vi "Get 4 Tables BY DP.vi"(0 "Air Pressure [psia]":dbl, 3 "Dew Point [DegF]":dbl) -> (1 "Pressure Z":dbl=53.278814892593125, 4 "DP Z":dbl, 5 "HP Higher DP Psych Table":dbl[][](array[numeric])=[[6500.0, 11.55684946, 0.0, 0.0, 0.0, 0.0, 0.0, 0.0, 0.0, 5.0], [6500.0, 11.55684946, 5.0, 5.0, 100.0, 0.001292913, 9.050389509, 14.92783844, 2.574650733, 5.0], [6500.0, 11.55684946, 10.0, 8.763538956, 77.60281671, 0.001292913, 9.050389509, 15.08846683, 3.777521, 5.0], [6500.0, 11.55684946, 15.0, 12.36490821, 60.54642502, 0.001292913, 9.050389509, 15.24909521, 4.980391266, 5.0], [6500.0, 11.55684946, 20.0, 15.80209708, 47.4855805, 0.001292913, 9.050389509, 15.4097236, 6.183261533, 5.0], [6500.0, 11.55684946, 25.0, 19.0756876, 37.43077436, 0.001292913, 9.050389509, 15.57035199, 7.386131799, 5.0], [6500.0, 11.55684946, 30.0, 22.18850798, 29.64995401, 0.001292913, 9.050389509, 15.73098037, 8.589002065, 5.0], [6500.0, 11.55684946, 35.0, 25.14521247, 23.98042946, 0.001292913, 9.050389509, 15.89160876, 9.791872332, 5.0], [6500.0, 11.55684946, 40.0, 27.95183421, 19.69610149, 0.001292913, 9.050389509, 16.05223714, 10.9947426, 5.0], [6500.0, 11.55684946, 45.0, 30.61535932, 16.2482458, 0.001292913, 9.050389509, 16.21286553, 12.19761286, 5.0], [6500.0, 11.55684946, 50.0, 33.21581881, 13.4609987, 0.001292913, 9.050389509, 16.37349392, 13.40048313, 5.0], [6500.0, 11.55684946, 55.0, 35.78456941, 11.19790107, 0.001292913, 9.050389509, 16.5341223, 14.6033534, 5.0], [6500.0, 11.55684946, 60.0, 38.24289128, 9.352562028, 0.001292913, 9.050389509, 16.69475069, 15.80622366, 5.0], [6500.0, 11.55684946, 65.0, 40.59668627, 7.841647488, 0.001292913, 9.050389509, 16.85537907, 17.00909393, 5.0], [6500.0, 11.55684946, 70.0, 42.851757, 6.599588278, 0.001292913, 9.050389509, 17.01600746, 18.2119642, 5.0], [6500.0, 11.55684946, 75.0, 45.01373336, 5.574566408, 0.001292913, 9.050389509, 17.17663585, 19.41483446, 5.0], [6500.0, 11.55684946, 80.0, 47.08801848, 4.725456286, 0.001292913, 9.050389509, 17.33726423, 20.61770473, 5.0], [6500.0, 11.55684946, 85.0, 49.07976369, 4.019482866, 0.001292913, 9.050389509, 17.49789262, 21.820575, 5.0], [6500.0, 11.55684946, 90.0, 50.99384196, 3.430420591, 0.001292913, 9.050389509, 17.65852101, 23.02344526, 5.0], [6500.0, 11.55684946, 95.0, 52.83484458, 2.937202158, 0.001292913, 9.050389509, 17.81914939, 24.22631553, 5.0], [6500.0, 11.55684946, 100.0, 54.60708072, 2.522839263, 0.001292913, 9.050389509, 17.97977778, 25.42918579, 5.0], [6500.0, 11.55684946, 105.0, 56.31458155, 2.173581867, 0.001292913, 9.050389509, 18.14040616, 26.63205606, 5.0], [6500.0, 11.55684946, 110.0, 57.9611144, 1.878260621, 0.001292913, 9.050389509, 18.30103455, 27.83492633, 5.0], [6500.0, 11.55684946, 115.0, 59.55019028, 1.62777051, 0.001292913, 9.050389509, 18.46166294, 29.03779659, 5.0], [6500.0, 11.55684946, 120.0, 61.08508025, 1.414663823, 0.001292913, 9.050389509, 18.62229132, 30.24066686, 5.0]], 6 "HP Lower DP Psych Table":dbl[][](array[numeric])=[[6500.0, 11.55684946, 0.0, 8.36519e-16, 100.0, 0.000997316, 6.981212001, 14.76020634, 1.058152276, 0.0], [6500.0, 11.55684946, 5.0, 3.963707944, 77.17374703, 0.000997316, 6.981212001, 14.92075855, 2.260366318, 0.0], [6500.0, 11.55684946, 10.0, 7.771498018, 59.88900146, 0.000997316, 6.981212001, 15.08131075, 3.462580359, 0.0], [6500.0, 11.55684946, 15.0, 11.41785035, 46.72594488, 0.000997316, 6.981212001, 15.24186295, 4.664794401, 0.0], [6500.0, 11.55684946, 20.0, 14.90004443, 36.64640178, 0.000997316, 6.981212001, 15.40241516, 5.867008442, 0.0], [6500.0, 11.55684946, 25.0, 18.218017, 28.88673111, 0.000997316, 6.981212001, 15.56296736, 7.069222484, 0.0], [6500.0, 11.55684946, 30.0, 21.37405669, 22.8819805, 0.000997316, 6.981212001, 15.72351957, 8.271436525, 0.0], [6500.0, 11.55684946, 35.0, 24.37240393, 18.50659597, 0.000997316, 6.981212001, 15.88407177, 9.473650567, 0.0], [6500.0, 11.55684946, 40.0, 27.21878765, 15.20021954, 0.000997316, 6.981212001, 16.04462398, 10.67586461, 0.0], [6500.0, 11.55684946, 45.0, 29.9200054, 12.53938011, 0.000997316, 6.981212001, 16.20517618, 11.87807865, 0.0], [6500.0, 11.55684946, 50.0, 32.51301876, 10.38835708, 0.000997316, 6.981212001, 16.36572838, 13.08029269, 0.0], [6500.0, 11.55684946, 55.0, 35.11238388, 8.641839847, 0.000997316, 6.981212001, 16.52628059, 14.28250673, 0.0], [6500.0, 11.55684946, 60.0, 37.59965819, 7.217722561, 0.000997316, 6.981212001, 16.68683279, 15.48472077, 0.0], [6500.0, 11.55684946, 65.0, 39.98076757, 6.051693196, 0.000997316, 6.981212001, 16.847385, 16.68693482, 0.0], [6500.0, 11.55684946, 70.0, 42.26156139, 5.093149563, 0.000997316, 6.981212001, 17.0079372, 17.88914886, 0.0], [6500.0, 11.55684946, 75.0, 44.44773195, 4.302101778, 0.000997316, 6.981212001, 17.1684894, 19.0913629, 0.0], [6500.0, 11.55684946, 80.0, 46.54475421, 3.64681168, 0.000997316, 6.981212001, 17.32904161, 20.29357694, 0.0], [6500.0, 11.55684946, 85.0, 48.55785849, 3.101985539, 0.000997316, 6.981212001, 17.48959381, 21.49579098, 0.0], [6500.0, 11.55684946, 90.0, 50.49199835, 2.647384109, 0.000997316, 6.981212001, 17.65014602, 22.69800502, 0.0], [6500.0, 11.55684946, 95.0, 52.35184609, 2.266748963, 0.000997316, 6.981212001, 17.81069822, 23.90021906, 0.0], [6500.0, 11.55684946, 100.0, 54.14179034, 1.946969591, 0.000997316, 6.981212001, 17.97125043, 25.10243311, 0.0], [6500.0, 11.55684946, 105.0, 55.86593869, 1.677434572, 0.000997316, 6.981212001, 18.13180263, 26.30464715, 0.0], [6500.0, 11.55684946, 110.0, 57.52813184, 1.4495241, 0.000997316, 6.981212001, 18.29235483, 27.50686119, 0.0], [6500.0, 11.55684946, 115.0, 59.13194983, 1.256211495, 0.000997316, 6.981212001, 18.45290704, 28.70907523, 0.0], [6500.0, 11.55684946, 120.0, 60.6807286, 1.09174908, 0.000997316, 6.981212001, 18.61345924, 29.91128927, 0.0]], 7 "LP Higher DP Psych Table":dbl[][](array[numeric])=[[7000.0, 11.3399368, 0.0, 0.0, 0.0, 0.0, 0.0, 0.0, 0.0, 5.0], [7000.0, 11.3399368, 5.0, 5.0, 100.0, 0.001317696, 9.223874019, 15.21398618, 2.601001048, 5.0], [7000.0, 11.3399368, 10.0, 8.746163989, 77.60281671, 0.001317696, 9.223874019, 15.37769361, 3.803926334, 5.0], [7000.0, 11.3399368, 15.0, 12.32952445, 60.54642502, 0.001317696, 9.223874019, 15.54140104, 5.006851619, 5.0], [7000.0, 11.3399368, 20.0, 15.74835457, 47.4855805, 0.001317696, 9.223874019, 15.70510847, 6.209776905, 5.0], [7000.0, 11.3399368, 25.0, 19.0035042, 37.43077436, 0.001317696, 9.223874019, 15.8688159, 7.412702191, 5.0], [7000.0, 11.3399368, 30.0, 22.09803756, 29.64995401, 0.001317696, 9.223874019, 16.03252333, 8.615627477, 5.0], [7000.0, 11.3399368, 35.0, 25.03680586, 23.98042946, 0.001317696, 9.223874019, 16.19623076, 9.818552762, 5.0], [7000.0, 11.3399368, 40.0, 27.82599156, 19.69610149, 0.001317696, 9.223874019, 16.35993819, 11.02147805, 5.0], [7000.0, 11.3399368, 45.0, 30.47269553, 16.2482458, 0.001317696, 9.223874019, 16.52364561, 12.22440333, 5.0], [7000.0, 11.3399368, 50.0, 33.04717386, 13.4609987, 0.001317696, 9.223874019, 16.68735304, 13.42732862, 5.0], [7000.0, 11.3399368, 55.0, 35.59971499, 11.19790107, 0.001317696, 9.223874019, 16.85106047, 14.63025391, 5.0], [7000.0, 11.3399368, 60.0, 38.0423982, 9.352562028, 0.001317696, 9.223874019, 17.0147679, 15.83317919, 5.0], [7000.0, 11.3399368, 65.0, 40.38114501, 7.841647488, 0.001317696, 9.223874019, 17.17847533, 17.03610448, 5.0], [7000.0, 11.3399368, 70.0, 42.62176507, 6.599588278, 0.001317696, 9.223874019, 17.34218276, 18.23902976, 5.0], [7000.0, 11.3399368, 75.0, 44.76988541, 5.574566408, 0.001317696, 9.223874019, 17.50589019, 19.44195505, 5.0], [7000.0, 11.3399368, 80.0, 46.83089832, 4.725456286, 0.001317696, 9.223874019, 17.66959762, 20.64488033, 5.0], [7000.0, 11.3399368, 85.0, 48.80993978, 4.019482866, 0.001317696, 9.223874019, 17.83330504, 21.84780562, 5.0], [7000.0, 11.3399368, 90.0, 50.71186298, 3.430420591, 0.001317696, 9.223874019, 17.99701247, 23.05073091, 5.0], [7000.0, 11.3399368, 95.0, 52.5412371, 2.937202158, 0.001317696, 9.223874019, 18.1607199, 24.25365619, 5.0], [7000.0, 11.3399368, 100.0, 54.30234788, 2.522839263, 0.001317696, 9.223874019, 18.32442733, 25.45658148, 5.0], [7000.0, 11.3399368, 105.0, 55.99920198, 2.173581867, 0.001317696, 9.223874019, 18.48813476, 26.65950676, 5.0], [7000.0, 11.3399368, 110.0, 57.63554279, 1.878260621, 0.001317696, 9.223874019, 18.65184219, 27.86243205, 5.0], [7000.0, 11.3399368, 115.0, 59.21485727, 1.62777051, 0.001317696, 9.223874019, 18.81554962, 29.06535733, 5.0], [7000.0, 11.3399368, 120.0, 60.74039319, 1.414663823, 0.001317696, 9.223874019, 18.97925705, 30.26828262, 5.0]], 8 "LP Lower DP Psych Table":dbl[][](array[numeric])=[[7000.0, 11.3399368, 0.0, 8.33951e-16, 100.0, 0.001016424, 7.114968311, 15.04300403, 1.078425911, 0.0], [7000.0, 11.3399368, 5.0, 3.948335527, 77.17374703, 0.001016424, 7.114968311, 15.20663233, 2.280682372, 0.0], [7000.0, 11.3399368, 10.0, 7.739796261, 59.88900146, 0.001016424, 7.114968311, 15.37026063, 3.482938834, 0.0], [7000.0, 11.3399368, 15.0, 11.36912414, 46.72594488, 0.001016424, 7.114968311, 15.53388893, 4.685195295, 0.0], [7000.0, 11.3399368, 20.0, 14.83387104, 36.64640178, 0.001016424, 7.114968311, 15.69751723, 5.887451757, 0.0], [7000.0, 11.3399368, 25.0, 18.13423563, 28.88673111, 0.001016424, 7.114968311, 15.86114553, 7.089708218, 0.0], [7000.0, 11.3399368, 30.0, 21.27274225, 22.8819805, 0.001016424, 7.114968311, 16.02477382, 8.291964679, 0.0], [7000.0, 11.3399368, 35.0, 24.25382981, 18.50659597, 0.001016424, 7.114968311, 16.18840212, 9.494221141, 0.0], [7000.0, 11.3399368, 40.0, 27.0833859, 15.20021954, 0.001016424, 7.114968311, 16.35203042, 10.6964776, 0.0], [7000.0, 11.3399368, 45.0, 29.76832648, 12.53938011, 0.001016424, 7.114968311, 16.51565872, 11.89873406, 0.0], [7000.0, 11.3399368, 50.0, 32.33520359, 10.38835708, 0.001016424, 7.114968311, 16.67928702, 13.10099052, 0.0], [7000.0, 11.3399368, 55.0, 34.91879392, 8.641839847, 0.001016424, 7.114968311, 16.84291532, 14.30324699, 0.0], [7000.0, 11.3399368, 60.0, 37.39082596, 7.217722561, 0.001016424, 7.114968311, 17.00654362, 15.50550345, 0.0], [7000.0, 11.3399368, 65.0, 39.75724943, 6.051693196, 0.001016424, 7.114968311, 17.17017192, 16.70775991, 0.0], [7000.0, 11.3399368, 70.0, 42.02392458, 5.093149563, 0.001016424, 7.114968311, 17.33380022, 17.91001637, 0.0], [7000.0, 11.3399368, 75.0, 44.19654431, 4.302101778, 0.001016424, 7.114968311, 17.49742851, 19.11227283, 0.0], [7000.0, 11.3399368, 80.0, 46.28057565, 3.64681168, 0.001016424, 7.114968311, 17.66105681, 20.31452929, 0.0], [7000.0, 11.3399368, 85.0, 48.28123636, 3.101985539, 0.001016424, 7.114968311, 17.82468511, 21.51678575, 0.0], [7000.0, 11.3399368, 90.0, 50.20346246, 2.647384109, 0.001016424, 7.114968311, 17.98831341, 22.71904222, 0.0], [7000.0, 11.3399368, 95.0, 52.05190619, 2.266748963, 0.001016424, 7.114968311, 18.15194171, 23.92129868, 0.0], [7000.0, 11.3399368, 100.0, 53.83093448, 1.946969591, 0.001016424, 7.114968311, 18.31557001, 25.12355514, 0.0], [7000.0, 11.3399368, 105.0, 55.54463186, 1.677434572, 0.001016424, 7.114968311, 18.47919831, 26.3258116, 0.0], [7000.0, 11.3399368, 110.0, 57.19681648, 1.4495241, 0.001016424, 7.114968311, 18.64282661, 27.52806806, 0.0], [7000.0, 11.3399368, 115.0, 58.79104547, 1.256211495, 0.001016424, 7.114968311, 18.80645491, 28.73032452, 0.0], [7000.0, 11.3399368, 120.0, 60.33063248, 1.09174908, 0.001016424, 7.114968311, 18.9700832, 29.93258098, 0.0]])   [LabVIEW 2020]
panel:
  in  "DP Array":dbl[](array[numeric])=[0.0, 5.0, 10.0, 15.0, 20.0, 25.0, 30.0, 35.0, 40.0, 45.0, 50.0, 55.0, 60.0, 65.0, 70.0, 75.0, 80.0, 85.0, 90.0, 95.0, 100.0, 105.0, 110.0, 115.0, 120.0]
  in  "Pressure Array":dbl[](array[numeric])=[15.51026974, 15.23488864, 14.96348006, 14.696, 14.43240481, 14.17265118, 13.91669613, 13.66449702, 13.41601153, 13.17119769, 12.93001384, 12.69241866, 12.45837117, 12.22783068, 12.00075687, 11.77710969, 11.55684946, 11.3399368]
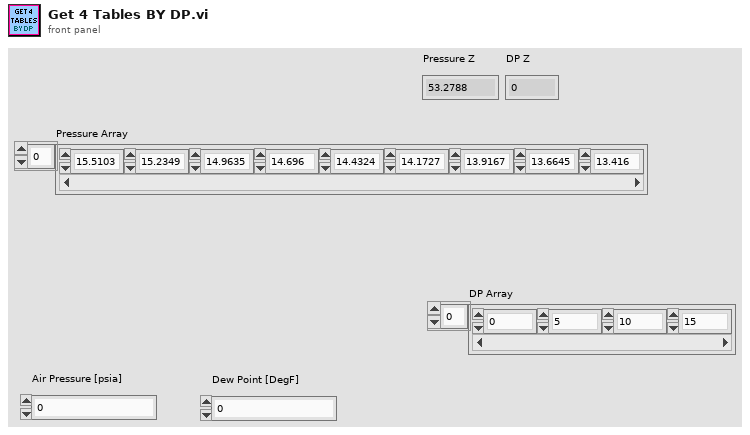
[diagram p1: front panel]
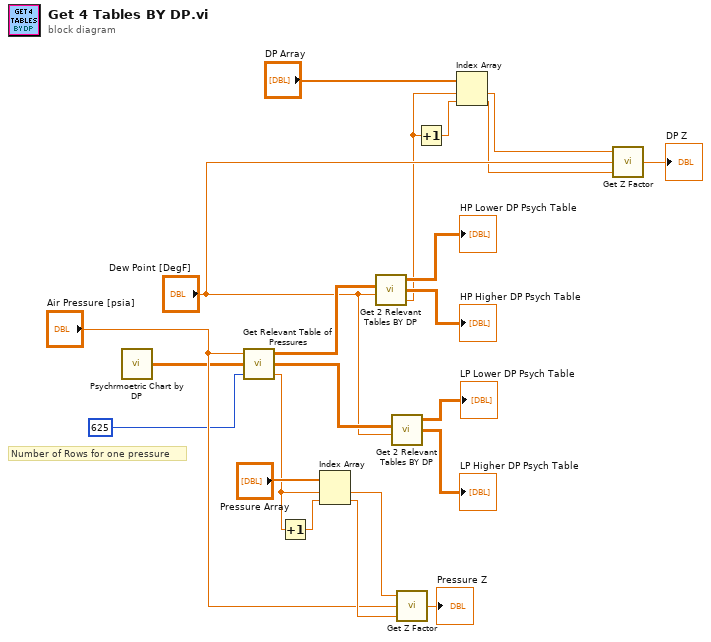
[diagram p0: block diagram]
diagram:
  # "Number of Rows for one pressure"
  n1 = call "Psychrmoetric Chart by DP.vi"() -> ("Psych Chart by DP"=w2:dbl[][])
  n2 = call "Get Relevant Table of Pressures.vi"("Length of List for 1 Pressure"=625 ("Length of List for a Single Pressure"), "Psych Table"=w2, "Air Pressure [psia]"="Air Pressure [psia]") -> ("Pressure Index"=w13:dbl, "Lower Pressure Psych Table"=w19:dbl[][], "Higher Pressure Psych Table"=w22:dbl[][])
  n3 = Increment(x=w13) -> (x+1=w12:dbl)
  n4 = Index Array(array="Pressure Array", index #1=w13, index #2=w12) -> (element #1=w11:dbl, element #2=w10:dbl)
  n5 = call "Get 2 Relevant Tables BY DP.vi"("Psych Table"=w22, "Dew Point [DegF]"="Dew Point [DegF]") -> ("Lower DP Psych Table"=→"HP Lower DP Psych Table":dbl[][], "Higher DP Psych Table"=→"HP Higher DP Psych Table":dbl[][], "DP Index"=w8:dbl)  [unwired: 4 in]
  n6 = call "Get 2 Relevant Tables BY DP.vi"("Psych Table"=w19, "Dew Point [DegF]"="Dew Point [DegF]") -> ("Lower DP Psych Table"=→"LP Lower DP Psych Table":dbl[][], "Higher DP Psych Table"=→"LP Higher DP Psych Table":dbl[][])  [unwired: 4 in, 1 out]
  n7 = call "Get Z Factor.vi"("X2"=w10, "Xi"="Air Pressure [psia]", "X1"=w11) -> ("Z"=→"Pressure Z":dbl)  [unwired: 2 in]
  n8 = Increment(x=w8) -> (x+1=w9:dbl)
  n9 = Index Array(array="DP Array", index #1=w8, index #2=w9) -> (element #1=w7:dbl, element #2=w6:dbl)
  n10 = call "Get Z Factor.vi"("X2"=w6, "Xi"="Dew Point [DegF]", "X1"=w7) -> ("Z"=→"DP Z":dbl)  [unwired: 2 in]
